vi "barrido.vi"(10 "File Path":path) -> (1 "ARREGLO DE SALIDA":string[](array[string]), 2 "Image":T1(plugin-control), 4 "size(s)":i32[](array[numeric]))   [LabVIEW 2016]
panel:
  out "size(s) 2":i32
  out "Array":string[](array[string])
  out "Image Pixels (U8)":u8[][](array[numeric])
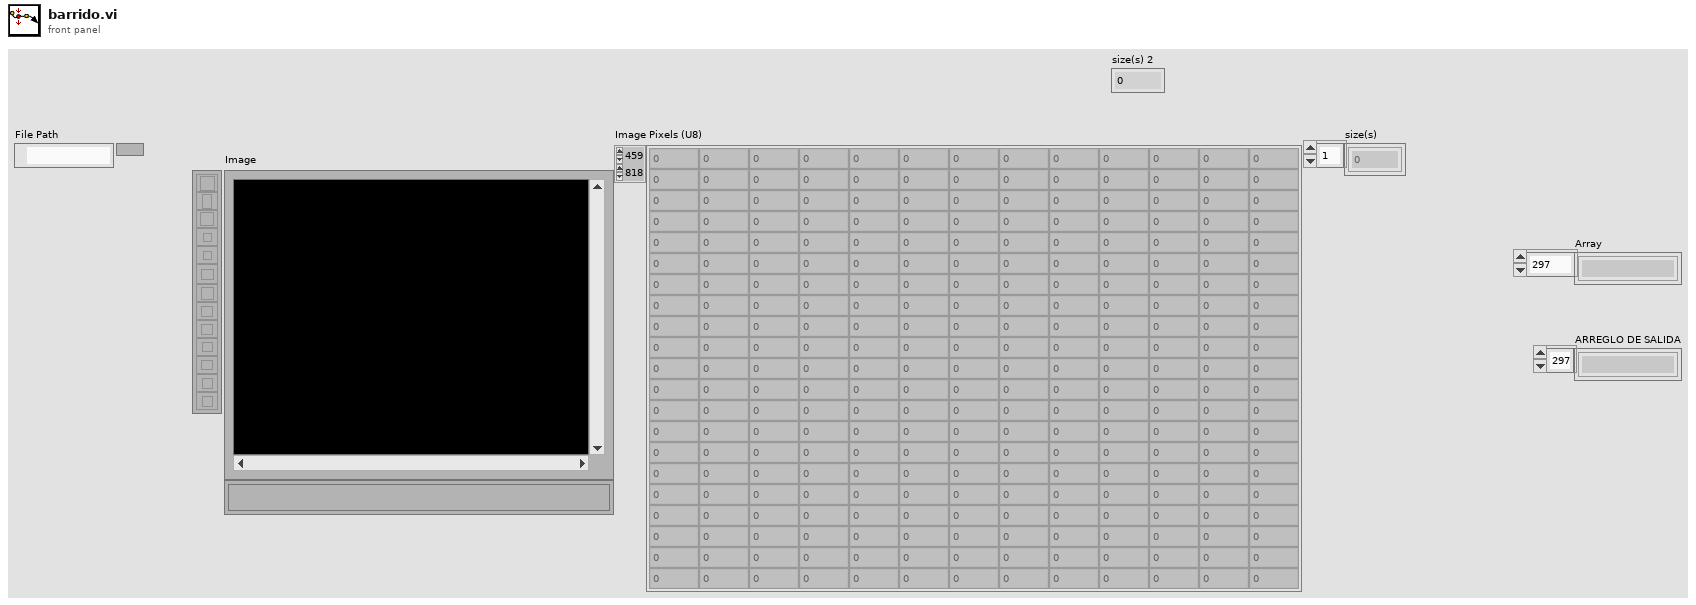
[diagram p1: front panel]
types:
  T1 = typedef "IMAQ Image.ctl" = refnum<image>
  T2 = cluster{"Global Rectangle":i32[], "Contours":cluster{"Contour Type":u32, "ROI Type":u32, "Points":i32[]}[]}
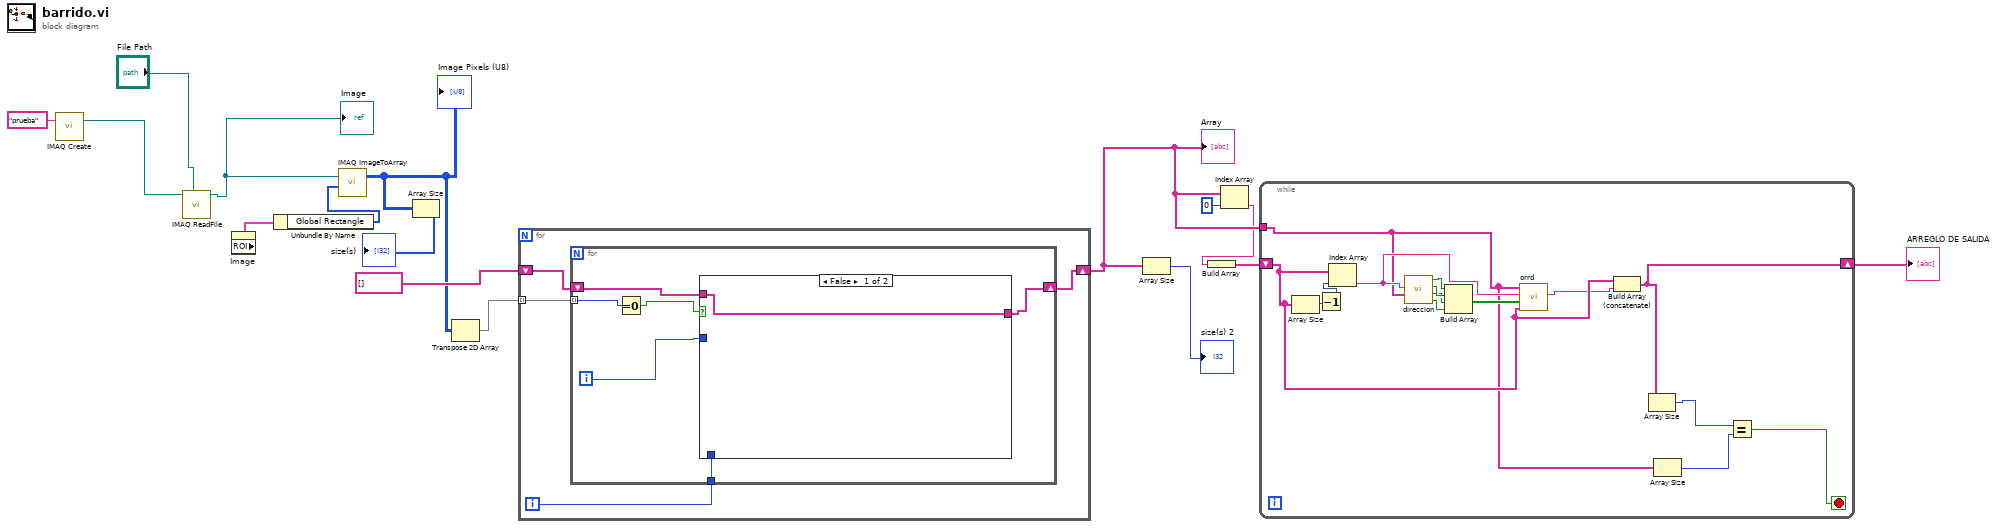
[diagram p0: block diagram]
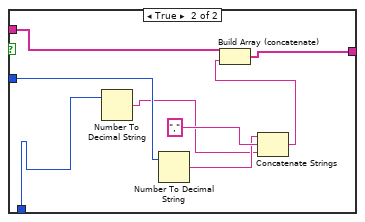
[diagram p2: hidden frame]
diagram:
  n1 = call "IMAQ Create"("Image Name"="prueba") -> ("New Image"=w16:T1)  [unwired: 4 in, 1 out]
  n2 = call "IMAQ ReadFile"("File Path"="File Path", "Image"=w16) -> ("Image Out"=w1:T1)  [unwired: 5 in, 4 out]
  "Image" <- w1
  n3 = property on="Image" class="ImageControl"() -> ("ROI"=w2:T2)  [unwired: 2 in, 2 out]
  n4 = Unbundle By Name(w2) -> ("Global Rectangle"=w9:i32[])
  n5 = call "IMAQ ImageToArray"("Optional Rectangle"=w9, "Image"=w1) -> ("Image Pixels (U8)"=w11:u8[][])  [unwired: 2 in, 4 out]
  "Image Pixels (U8)" <- w11
  n6 = Array Size(array=w11) -> (size(s)=→"size(s)":i32[])
  n7 = Transpose 2D Array(2D array=w11) -> (transposed array=w10:u8[][])
  n8 = for {
    tunnel: w10 -> [w20] mode=indexing
    shift-right: [w17] -> w7
    shift-left: string[] [] -> [w18]
    i -> [w19]
    n9 = for {
      tunnel: w20 -> [w26] mode=indexing
      tunnel: w19 -> [w24]
      shift-right: [w22] -> w17
      shift-left: w18 -> [w21]
      i -> [w23]
      n10 = Equal To 0?(x=w26) -> (x = 0?=w25:bool)
      n11 = case shown="False" w25 {
        tunnel: w24 -> [_ w35]
        tunnel: w23 -> [_ w33]
        tunnel: [w27 w30] -> w22
        tunnel: w21 -> [w27 w32]
        frame False {
        }
        frame True {
          n12 = Number To Decimal String(number=w35) -> (decimal integer string=w28:string)  [unwired: 1 in]
          n13 = Number To Decimal String(number=w33) -> (decimal integer string=w29:string)  [unwired: 1 in]
          n14 = Concatenate Strings(w29, "," ("string"), w28) -> (w31:string)
          n15 = Build Array (concatenate)(w32, w31) -> (w30:string[])
        }
      }
    }
  }
  "Array" <- w7
  n16 = Array Size(array=w7) -> (size(s)=→"size(s) 2":i32)
  n17 = Index Array(array=w7, index=0) -> (element=w4:string)
  n18 = Build Array(w4) -> (w5:string[])
  n19 = while {
    tunnel: w7 -> [w39]
    shift-right: [w40] -> w3
    shift-left: w5 -> [w42]
    stop <- w36 stop-if-true
    n20 = Array Size(array=w42) -> (size(s)=w49:i32)
    n21 = Decrement(x=w49) -> (x-1=w50:i32)
    n22 = Index Array(array=w42, index=w50) -> (element=w43:string)
    n23 = call "direccion.vi"("Array"=w39, "String"=w43) -> ("DERECHA"=w45:bool, "IZQUIERDA"=w46:bool, "ABAJO"=w47:bool, "ARRIBA"=w48:bool)  [unwired: 6 in]
    n24 = Build Array(w48, w47, w46, w45) -> (w44:bool[])
    n25 = call "orrd.vi"("arreglo modificado"=w42, "Arreglo dim"=w44, "entrada"=w43, "arreglo entrada"=w39) -> ("salida"=w41:string)  [unwired: 7 in]
    n26 = Build Array (concatenate)(w42, w41) -> (w40:string[])
    n27 = Array Size(array=w40) -> (size(s)=w38:i32)
    n28 = Array Size(array=w39) -> (size(s)=w37:i32)
    n29 = Equal?(x=w38, y=w37) -> (x = y?=w36:bool)
  }
  "ARREGLO DE SALIDA" <- w3
